vi "Prova reserve chassis.vi"() -> ()   [LabVIEW 2019]
panel:
  in  "stop":bool
  out "error out 2":errorcluster
  out "error out":errorcluster
  in  "device in 2":tag
  in  "unreserve":bool
  in  "reserve":bool
  in  "device in":tag
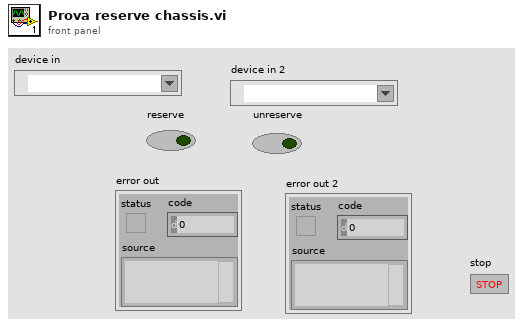
[diagram p1: front panel]
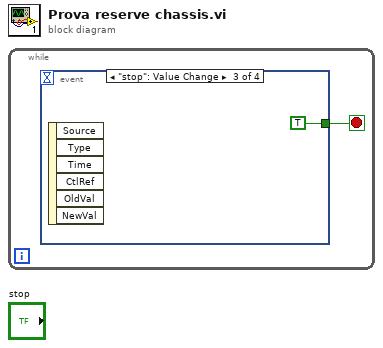
[diagram p0: block diagram]
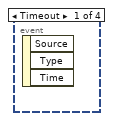
[diagram p2: hidden frame]
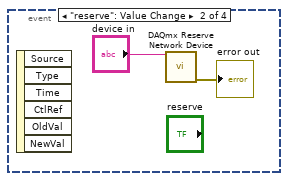
[diagram p3: hidden frame]
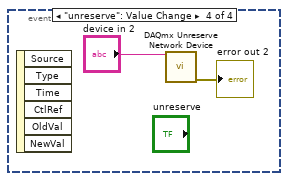
[diagram p4: hidden frame]
diagram:
  n1 = while {
    stop <- w1 stop-if-true
    n2 = event shown="[2] \"stop\": Value Change" {
      selector: _ -> [_ _ _ _]
      dyn-events: _ -> [_ _ _ _]
      timeout: _ -> [_ _ _ _]
      tunnel: [_ _ TRUE _] -> w1
      event Timeout {
        n3 = event-data() -> ()  [unwired: 1 in, 3 out]
      }
      event "reserve": Value Change {
        n4 = event-data() -> ()  [unwired: 1 in, 6 out]
        n5 = call <vilib>:"DAQmx Reserve Network Device.vi"("device in"="device in") -> ("error out"=→"error out":errorcluster)  [unwired: 13 in, 1 out]
      }
      event "stop": Value Change {
        n6 = event-data() -> ()  [unwired: 1 in, 6 out]
      }
      event "unreserve": Value Change {
        n7 = event-data() -> ()  [unwired: 1 in, 6 out]
        n8 = call <vilib>:"DAQmx Unreserve Network Device.vi"("device in"="device in 2") -> ("error out"=→"error out 2":errorcluster)  [unwired: 13 in, 1 out]
      }
    }
  }
